vi "Initialize.vi"(8 "error in (no error)":errorcluster, 11 "device data model in":refnum<class "ELAN Data Model.lvclass">) -> (0 "error out":errorcluster, 3 "device data model out":refnum<class "ELAN Data Model.lvclass">)   [LabVIEW 2021, in "ELAN Data Model.lvclass"]
doc: "This VI initializes the device data model."
uses:
  ELAN Data Model.lvclass
  Type Definitions/Data Model.ctl
  Type Definitions/Value full.ctl
  Data Unit/ELAN PC Data Unit/Elan units.ctl
  Data Unit/ELAN PC Data Unit/Elan measured variable.ctl
  Data Unit/ELAN PC Data Unit/Elan channel state.ctl
  ELAN Data Model.lvclass/ELAN Data Model.ctl
  Modbus_v121c/Data Model/Device Data Model.lvclass
  Data Unit/ELAN PC Data Unit/ELAN PDU.lvclass
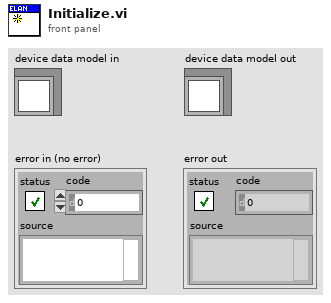
[diagram p1: front panel]
types:
  T1 = typedef "ELAN Data Model.lvclass/Data Model.ctl" = cluster{"UTC":u64, "Value":T2[]}
  T2 = typedef "ELAN Data Model.lvclass/Value full.ctl" = cluster{"Value":cluster{"Value":sgl, "units":T3, "component":T4}, "channel state":T5, "collective state":errorcluster}
  T3 = typedef "ELAN PDU.lvclass/Elan units.ctl" = enum16{"Invalid", "no dimension", "ppm", "ppb", "vpm", "ppm C1", "ppm C3", "ppm C6", "mg C/m3", "mg/m3", "%", "% vol", "% of measuring range", "% saturation", "%/°C", "%/K", "% weight", "mV/pH", "mV/mbar", "nA/mbar", "S/m", "S/cm", "mS/m", "mS/cm", "ìS/m", "ìS/cm", "S", "min", "H", "Pa", "MA", "uV", "MV", "V", "mbar", "hPa", "Ml/min", "kOhm", "MOhm", "S1", "°C", "Hz", "pH", "ug/l", "mg/l", "l/min", "uA", "mg/dm3", "kPa", "kOhm*cm", "MOhm*cm", "°", "1/min", "1/m", "g/m3", "g/l", "% Vol C"}
  T4 = typedef "ELAN PDU.lvclass/Elan measured variable.ctl" = enum16{"Invalid", "no component", "CO", "CO2", "CH4 (Methan)", "C6H14 (Hexan)", "SO2", "NO", "NO2", "CHClF2 (R22)", "C3H8 (Propan)", "C4H10 (Butan)", "O2", "C5H12 (Pentan)", "CnHm (THC)", "P (process pressure)", "pH", "T (temperature)", "C2H4 (Ethen)", "C2H2 (Ethin)", "C3H6 (Propen)", "C4H6", "C4H8", "C2H6", "NH3 (Ammoniak)", "N2O", "C6H6 (Benzol)", "SF6", "CH3OH (Methanol)", "C2H5OH (Ethanol)", "CH2Cl2", "C2H4Cl2", "CH3Cl", "C2H4O", "H2O (water vapor)", "G/l (conductivity)", "C", "S", "N", "CF4", "COCl2 (phosgene)", "CHF3 (R23)", "C2F6 (R116)", "------ (self defined component)", "C2H3Cl", "H2 (Hydrogen)", "Ar", "He", "Cl2", "N2"}
  T5 = typedef "ELAN PDU.lvclass/Elan channel state.ctl" = enum16{"Invalid", "Warm-up", "Pause", "Standby", "Measure", "Zero calibration", "Adjust component slope", "Not yet defined1", "Adjust curve dip", "Adjust linearization sensitivity", "Adjust temperature compensation", "Adjust pressure compensation", "Adjust linearization zero", "Not yet defined2", "Autocal", "Adjust phase", "Zero calibration of O2 sensor", "Synchronous zero calibration", "Purging for synchronous zero calibration", "Adjust analog output", "Adjust analog input", "Autocal check"}
  T6 = typedef "Device Data Model.lvclass/N channel.ctl" = cluster{"N DI channel":i32, "N DO channel":i32, "N AI channel":i32, "N AO channel":i32}
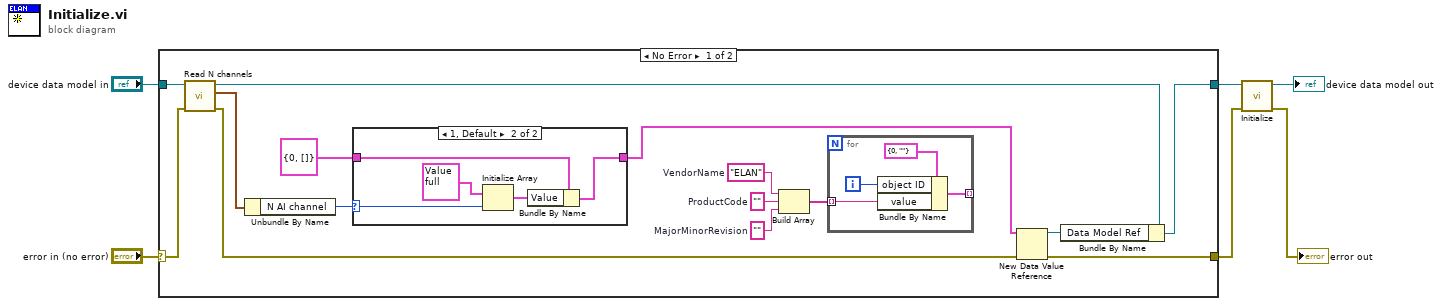
[diagram p0: block diagram]
diagram:
  n1 = case shown="No Error" "error in (no error)" {
    selector: "error in (no error)" -> [w12 w32]
    tunnel: "device data model in" -> [w13 w33]
    tunnel: [w15 w32] -> w5
    tunnel: [w17 w33] -> w4
    frame No Error {
      w19 = ""  # MajorMinorRevision
      w21 = ""  # ProductCode
      w20 = "ELAN"  # VendorName
      n2 = call-dynamic "Read N channels.vi"("error in (no error)"=w12, "device data model in"=w13) -> ("error out"=w11:errorcluster, "N channel"=w9:T6, "device data model out"=w14:refnum<class "ELAN Data Model.lvclass">)  [unwired: 7 in]
      n3 = Unbundle By Name(w9) -> ("N AI channel"=w10:i32)
      n4 = case shown="1, Default" w10 {
        selector: w10 -> [_ w24]
        tunnel: T1 {"UTC"=0, "Value"=[]} ("Data Model") -> [w22 w27]
        tunnel: [w22 w25] -> w7
        frame 0 {
        }
        frame 1, Default {
          n5 = Initialize Array(T2 {"Value"={"Value"=0.0, "units"=enum."Invalid", "component"=enum."Invalid"}, "channel state"=enum."Invalid", "collective state"={"status"=FALSE, "code"=0, "source"=""}} ("Value full"), w24) -> (w26:T2[])
          n6 = Bundle By Name(cluster=w27, "Value"=w26) -> (w25:T1)
        }
      }
      n7 = Build Array(w20, w21, w19) -> (w18:string[])
      n8 = for {
        tunnel: w18 -> [w29] mode=indexing
        tunnel: [w28] -> _ mode=indexing
        i -> [w30]
        n9 = Bundle By Name(cluster=cluster{"object ID":u8, "value":string} {"object ID"=0, "value"=""} ("Cluster"), "object ID"=w30, "value"=w29) -> (w28:cluster{"object ID":u8, "value":string})
      }
      n10 = New Data Value Reference(data value=w7, error in=w11) -> (data value reference=w16:refnum<data-value>, error out=w15:errorcluster)
      n11 = Bundle By Name(cluster=w14, "Data Model Ref"=w16) -> (w17:refnum<class "ELAN Data Model.lvclass">)
    }
    frame Error {
    }
  }
  n12 = call-parent "Initialize.vi"("error in"=w5, "device data model in"=w4) -> ("error out"=→"error out":errorcluster, "device data model out"=→"device data model out":refnum<class "ELAN Data Model.lvclass">)  [unwired: 8 in]
